vi "C37 Get Digital Configuration.vi"(8 "error in (no error)":errorcluster, 9 "Digital Index":i32, 10 "PMU Index":i32, 11 "Pseudo PDC ID":i32) -> (0 "error out":errorcluster, 2 "Channel Name":string, 3 "Digital Configuration":cluster{"normalBit":u8, "isValidBit":u8})   [LabVIEW 2017, in "C37118-DLL.lvlib"]
uses:
  C37118-DLL.lvlib
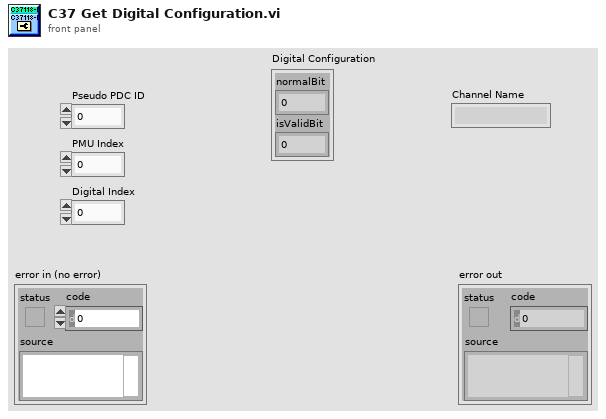
[diagram p1: front panel]
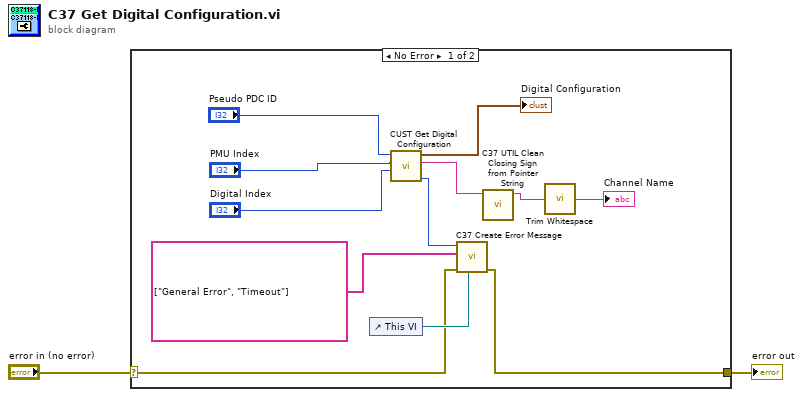
[diagram p0: block diagram]
diagram:
  n1 = case shown="No Error" "error in (no error)" {
    selector: "error in (no error)" -> [w13 w15]
    tunnel: [w12 w15] -> w2
    frame No Error {
      n2 = control-ref of="This VI"() -> (w14:refnum<vi>)
      n3 = call "CUST Get Digital Configuration.vi"("digitalIndex"="Digital Index", "pmuIndex"="PMU Index", "pseudoPdcId"="Pseudo PDC ID") -> ("function return"=w3:i32, "name out"=w4:string, "digitalCfg out"=→"Digital Configuration":cluster{"normalBit":u8, "isValidBit":u8})  [unwired: 6 in]
      n4 = call "C37 Create Error Message.vi"("VI Reference"=w14, "error in (no error)"=w13, "Error Messages"=string[] ["General Error", "Timeout"], "function return"=w3) -> ("error out"=w12:errorcluster)  [unwired: 7 in]
      n5 = call "C37 UTIL Clean Closing Sign from Pointer String.vi"("String In"=w4) -> ("String Out"=w9:string)  [unwired: 10 in]
      n6 = call <vilib>:"Trim Whitespace.vi"("string"=w9) -> ("trimmed string"=→"Channel Name":string)  [unwired: 1 in]
    }
    frame Error {
    }
  }
  "error out" <- w2
